vi "_Queue Last Ack.vi"(10 "Queue jettl":refnum<class "Queue jettl.lvclass">) -> (3 "Queue Last Ack Msg Strategy out":refnum<class "Queue Last Ack Msg Strategy.lvclass">)   [LabVIEW 2021, in "jettl.lvlib" / "jettl Msg Queue Last Ack.lvlib"]
uses:
  jettl Msg Queue Last Ack.lvlib
  Queue Last Ack Msg Strategy/Queue Last Ack Msg Strategy.lvclass
  Queue jettl/Queue jettl.lvclass
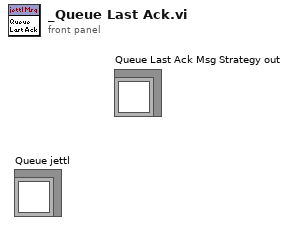
[diagram p1: front panel]
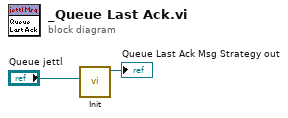
[diagram p0: block diagram]
diagram:
  n1 = call "Init.vi"("Queue jettl"="Queue jettl") -> ("Queue Last Ack Msg Strategy out"=→"Queue Last Ack Msg Strategy out":refnum<class "Queue Last Ack Msg Strategy.lvclass">)  [unwired: 10 in]
